vi "Transformations.vi"(2 "error in (no error)":errorcluster, 3 "Level data":cluster{"ori_X":dbl, "ori_Y":dbl, "ori_Z":dbl}, 4 "Initial Orentation":T1, 5 "SceneObject in":refnum<vi>) -> (0 "error out":errorcluster, 1 "SceneObject out":refnum<vi>)   [LabVIEW 2014]
doc: "Applies the rotational transformations needed to represent the smartphone motion. The level data is given as input to this task"
uses:
  <vilib>/picture/3D Picture Control/NI_3D Picture Control.lvlib
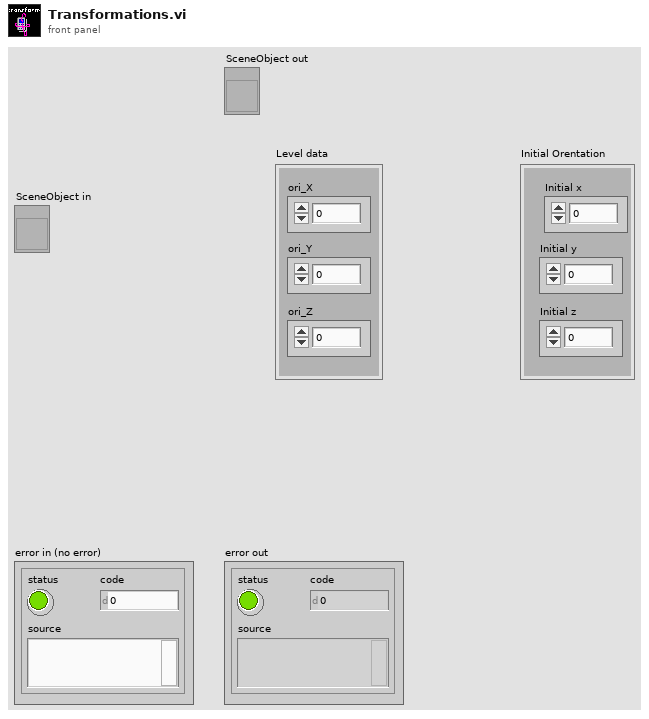
[diagram p1: front panel]
types:
  T1 = cluster{"Initial x":dbl, "Initial y":dbl, "Initial z":dbl}
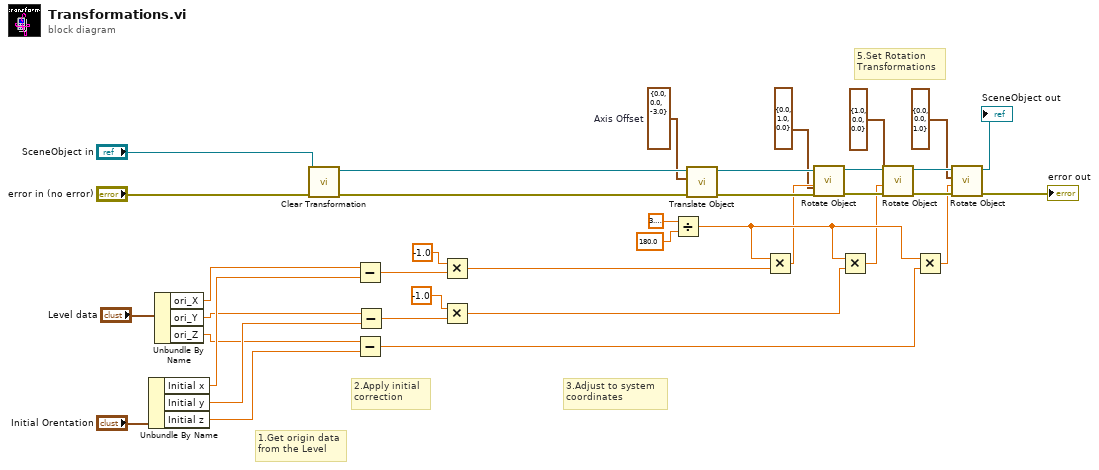
[diagram p0: block diagram]
diagram:
  w29 = cluster{"X":sgl, "Y":sgl, "Z":sgl} {"X"=0.0, "Y"=0.0, "Z"=-3.0}  # Axis Offset
  # "5.Set Rotation \nTransformations"
  # "3.Adjust to system \ncoordinates"
  # "2.Apply initial \ncorrection"
  # "1.Get origin data\nfrom the Level"
  n1 = Unbundle By Name("Initial Orentation") -> ("Initial x"=w7:dbl, "Initial y"=w5:dbl, "Initial z"=w3:dbl)
  n2 = Unbundle By Name("Level data") -> ("ori_X"=w8:dbl, "ori_Y"=w6:dbl, "ori_Z"=w4:dbl)
  n3 = call <vilib>:"Clear Transformation.vi"("error in (no error)"="error in (no error)", "Object Refnum In"="SceneObject in") -> ("error out"=w31:errorcluster, "Object Refnum Out"=w34:refnum<vi>)  [unwired: 8 in]
  n4 = Subtract(x=w8, y=w7) -> (x-y=w24:dbl)
  n5 = Subtract(x=w4, y=w3) -> (x-y=w17:dbl)
  n6 = Subtract(x=w6, y=w5) -> (x-y=w2:dbl)
  n7 = Multiply(x=-1.0, y=w24) -> (x*y=w21:dbl)
  n8 = Multiply(x=-1.0 ("y"), y=w2) -> (x*y=w18:dbl)
  n9 = Divide(x=3.141592653589793, y=180.0) -> (x/y=w22:dbl)
  n10 = call <vilib>:"Translate Object.vi"("error in (no error)"=w31, "Translation"=w29, "Scene.Object In"=w34) -> ("error out"=w32:errorcluster, "Scene.Object Out"=w33:refnum<vi>)  [unwired: 7 in]
  n11 = Multiply(x=w22, y=w21) -> (x*y=w20:dbl)
  n12 = call <vilib>:"Rotate Object.vi"("error in (no error)"=w32, "Angle"=w20, "Axis"=cluster{"X":sgl, "Y":sgl, "Z":sgl} {"X"=0.0, "Y"=1.0, "Z"=0.0}, "Scene.Object In"=w33) -> ("error out"=w27:errorcluster, "Scene.Object Out"=w25:refnum<vi>)  [unwired: 6 in]
  n13 = Multiply(x=w22, y=w18) -> (x*y=w19:dbl)
  n14 = call <vilib>:"Rotate Object.vi"("error in (no error)"=w27, "Angle"=w19, "Axis"=cluster{"X":sgl, "Y":sgl, "Z":sgl} {"X"=1.0, "Y"=0.0, "Z"=0.0}, "Scene.Object In"=w25) -> ("error out"=w28:errorcluster, "Scene.Object Out"=w26:refnum<vi>)  [unwired: 6 in]
  n15 = Multiply(x=w22, y=w17) -> (x*y=w15:dbl)
  n16 = call <vilib>:"Rotate Object.vi"("error in (no error)"=w28, "Angle"=w15, "Axis"=cluster{"X":sgl, "Y":sgl, "Z":sgl} {"X"=0.0, "Y"=0.0, "Z"=1.0}, "Scene.Object In"=w26) -> ("error out"=→"error out":errorcluster, "Scene.Object Out"=→"SceneObject out":refnum<vi>)  [unwired: 6 in]
